vi "TDTRX6-Read Input Buffers.vi"(0 "RPcox":refnum<k7>, 5 "Next Buffer":i32, 7 "Pts Per Read":i32, 9 "AI Channels":i32[](array[numeric])=[1, 2], 11 "error in (no error)":errorcluster, 12 "#inputs":i32) -> (8 "Input array":dbl[][](array[numeric]), 15 "error out":errorcluster)   [LabVIEW 2020]
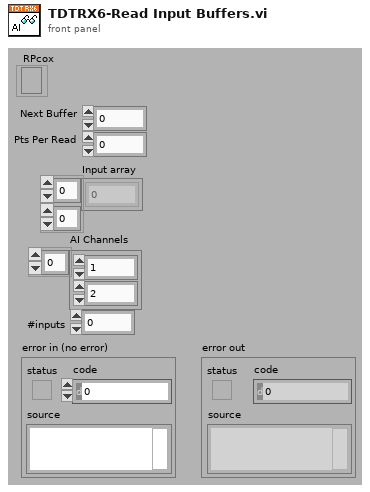
[diagram p1: front panel]
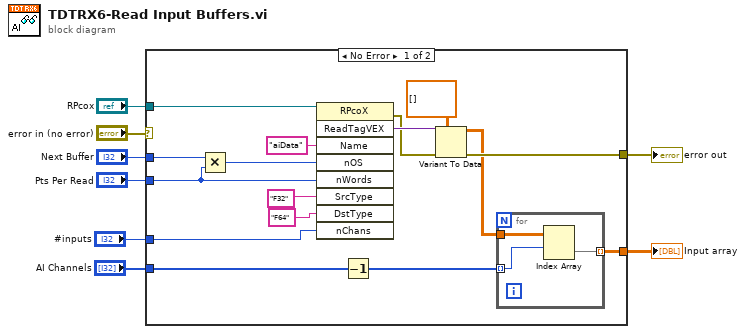
[diagram p0: block diagram]
diagram:
  n1 = case shown="No Error" "error in (no error)" {
    selector: "error in (no error)" -> [_ w28]
    tunnel: "Next Buffer" -> [w24 _]
    tunnel: "RPcox" -> [w23 _]
    tunnel: [w22 w28] -> w5
    tunnel: "Pts Per Read" -> [w14 _]
    tunnel: [w13 _] -> w3
    tunnel: "AI Channels" -> [w12 _]
    tunnel: "#inputs" -> [w11 _]
    frame No Error {
      n2 = Multiply(x=w24, y=w14) -> (x*y=w15:i32)
      n3 = invoke class="RPcoX" method="ReadTagVEX"(reference=w23, "Name"="aiData", "nOS"=w15, "nWords"=w14, "SrcType"="F32" ("DstType"), "DstType"="F64", "nChans"=w11) -> (error out=w17:errorcluster, "ReadTagVEX"=w20:variant)  [unwired: 2 in, 7 out]
      n4 = Decrement(x=w12) -> (x-1=w9:i32[])
      n5 = Variant To Data(error in=w17, type=dbl[][] [] ("Input array"), Variant=w20) -> (data=w10:dbl[][], error out=w22:errorcluster)
      n6 = for {
        tunnel: w10 -> [w27]
        tunnel: [w26] -> w13 mode=indexing
        tunnel: w9 -> [w25] mode=indexing
        n7 = Index Array(array=w27, index (row)=w25) -> (element=w26:dbl[])  [unwired: 1 in]
      }
    }
    frame Error {
    }
  }
  "Input array" <- w3
  "error out" <- w5
